vi "PUBLISH.vi"(0 "TCP session out":refnum<k5>, 5 "Channel":string, 7 "Message":string, 11 "error in":errorcluster) -> (4 "TCP session out":refnum<k5>, 6 "Data":T1, 15 "error out":errorcluster)   [LabVIEW 2023]
uses:
  SubVIs/Controls/redis-data.ctl
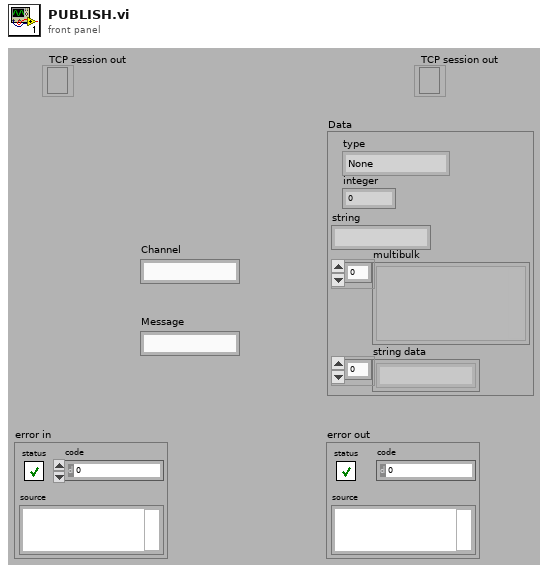
[diagram p1: front panel]
types:
  T1 = typedef "redis-data.ctl" = cluster{"type":enum16{"None", "Error", "Status", "Nil", "Integer", "String", "Multibulk"}, "integer":i64, "string":string, "multibulk":variant[], "string data":string[]}
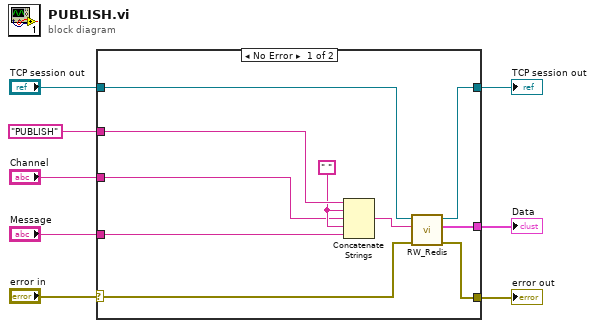
[diagram p0: block diagram]
diagram:
  n1 = case shown="No Error" "error in" {
    selector: "error in" -> [w17 w20]
    tunnel: "PUBLISH" -> [w14 _]
    tunnel: "TCP session out" -> [w10 w19]
    tunnel: [w16 w20] -> w6
    tunnel: [w15 _] -> w2
    tunnel: "Channel" -> [w12 _]
    tunnel: "Message" -> [w11 _]
    tunnel: [w9 w19] -> w1
    frame No Error {
      w13 = " "
      n2 = Concatenate Strings(w14, w13, w12, w13, w11) -> (w18:string)
      n3 = call "RW_Redis.vi"("error in"=w17, "command"=w18, "TCP session in"=w10) -> ("error out"=w16:errorcluster, "Data"=w15:T1, "TCP session out"=w9:refnum<k5>)  [unwired: 6 in]
    }
    frame Error {
    }
  }
  "error out" <- w6
  "TCP session out" <- w1
  "Data" <- w2
